vi "Log Event.vi"(8 "Event":string, 9 "Enum":enum16{"Information", "Warning", "Error"}(ring), 10 "Process":string, 11 "Log Refnum":refnum<vi>) -> ()   [LabVIEW 2015]
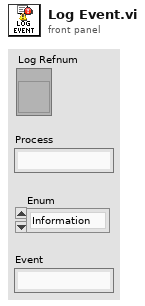
[diagram p1: front panel]
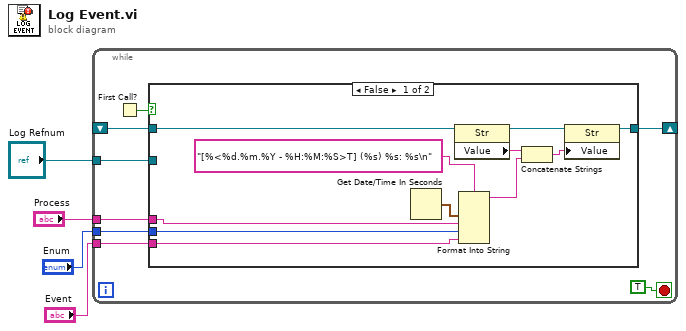
[diagram p0: block diagram]
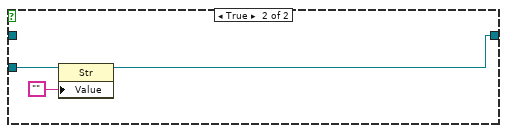
[diagram p2: hidden frame]
diagram:
  n1 = while {
    tunnel: "Log Refnum" -> [w11]
    shift-right: [w8] -> _
    shift-left: _ -> [w9]
    tunnel: "Process" -> [w7]
    tunnel: "Event" -> [w5]
    tunnel: "Enum" -> [w6]
    stop <- TRUE stop-if-true
    n2 = First Call?() -> (First Call?: T/F=w12:bool)
    n3 = case shown="False" w12 {
      tunnel: w11 -> [_ w26]
      tunnel: [w18 w24] -> w8
      tunnel: w9 -> [w17 _]
      tunnel: w7 -> [w15 _]
      tunnel: w6 -> [w14 _]
      tunnel: w5 -> [w13 _]
      frame False {
        n4 = Get Date/Time In Seconds() -> (seconds since 1Jan1904=w23:timestamp)
        n5 = property class="Str"(reference=w17) -> (reference out=w22:refnum<vi>, "Value"=w19:string)  [unwired: 1 in, 1 out]
        n6 = Format Into String(format string="[%<%d.%m.%Y - %H:%M:%S>T] (%s) %s: %s\n", w23, w15, w14, w13) -> (resulting string=w21:string)  [unwired: 2 in, 1 out]
        n7 = Concatenate Strings(w19, w21) -> (w20:string)
        n8 = property class="Str"(reference=w22, "Value"=w20) -> (reference out=w18:refnum<vi>)  [unwired: 1 in, 1 out]
      }
      frame True {
        n9 = property class="Str"(reference=w26, "Value"="") -> (reference out=w24:refnum<vi>)  [unwired: 1 in, 1 out]
      }
    }
  }
